vi "MU Mt Sync Calculate Position.vi"(4 "Continuous (F)":bool, 5 "Calibration Unit":u32, 6 "resolution":u64, 7 "MtTrackOffset":u8, 8 "error in (no error)":errorcluster, 9 "Samples":u64, 10 "SyncData":T1(array[cluster]), 11 "mtSyncHandle":T2) -> (0 "error out":errorcluster, 2 "MT_Position":dbl[](array[numeric]), 3 "Return Value":u64)   [LabVIEW 2017, in "MU_3SL_interface.lvlib"]
uses:
  MU_3SL_interface.lvlib
  handles/mtSyncHandle.ctl
  lib/MU_3SL_interface.dll
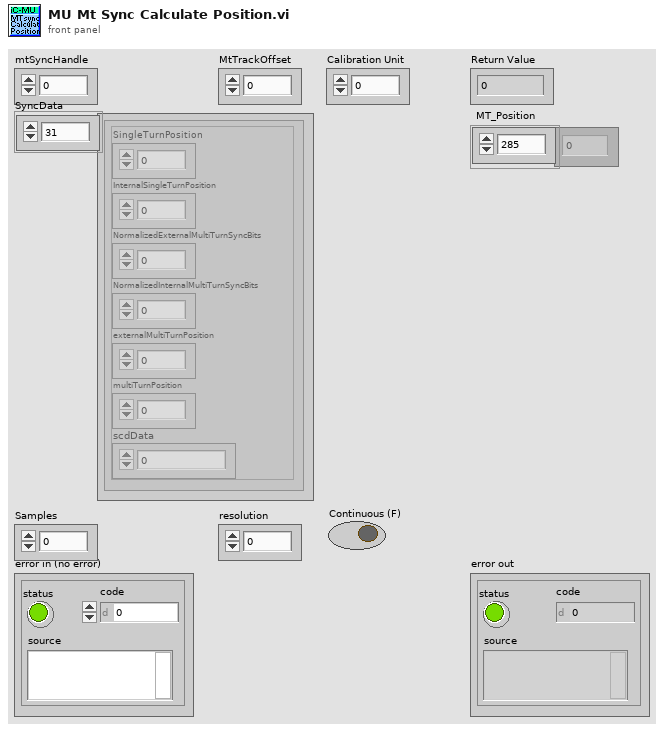
[diagram p1: front panel]
types:
  T1 = cluster{"SingleTurnPosition":u32, "InternalSingleTurnPosition":u32, "NormalizedExternalMultiTurnSyncBits":u32, "NormalizedInternalMultiTurnSyncBits":u32, "externalMultiTurnPosition":u32, "multiTurnPosition":u32, "scdData":u64}[]
  T2 = typedef "MU_3SL_interface.lvlib/mtSyncHandle.ctl" = u64
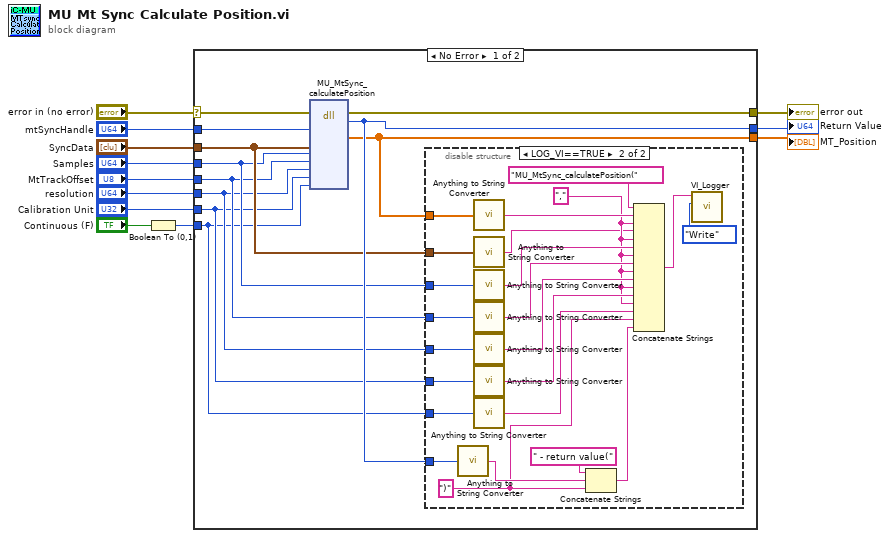
[diagram p0: block diagram]
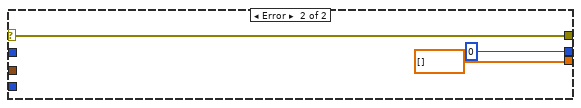
[diagram p3: hidden frame]
diagram:
  n1 = Boolean To (0,1)(Boolean="Continuous (F)") -> (0, 1=w4:i16)
  n2 = case shown="No Error" "error in (no error)" {
    selector: "error in (no error)" -> [w23 w49]
    tunnel: [w22 u64 0 ("Return Value")] -> w8
    tunnel: [w21 w49] -> w12
    tunnel: "mtSyncHandle" -> [w20 _]
    tunnel: [w19 dbl[] [] ("MT_OffsetError")] -> w9
    tunnel: "SyncData" -> [w18 _]
    tunnel: "Samples" -> [w17 _]
    tunnel: w4 -> [w13 _]
    tunnel: "resolution" -> [w15 _]
    tunnel: "MtTrackOffset" -> [w16 _]
    tunnel: "Calibration Unit" -> [w14 _]
    frame No Error {
      n3 = dll-call lib="C:/Users/bes/AppData/Roaming/work/mu_9so/icsubmodules/soft_mu_3sl_master/lv_interface/lib/MU_3SL_interface**.*" fn="MU_MtSync_calculatePosition"(error in=w23, "mtSyncHandle"=w20, "SynchronisationData"=w18, "numberOfSamples"=w17, "MtTrackOffset"=w16, "resolution"=w15, "Calibration Unit"=w14, "continuous"=w13) -> (error out=w21:errorcluster, "Return Value"=w22:u64, "MT_Position"=w19:dbl[])  [unwired: 10 in, 1 out]
      n4 = disable-structure shown="LOG_VI==TRUE" {
        disable-tunnel: w22 -> [_ w38]
        disable-tunnel: w19 -> [_ w42]
        disable-tunnel: w18 -> [_ w25]
        disable-tunnel: w17 -> [_ w40]
        disable-tunnel: w16 -> [_ w39]
        disable-tunnel: w15 -> [_ w36]
        disable-tunnel: w14 -> [_ w35]
        disable-tunnel: w13 -> [_ w34]
        frame condition #0 {
        }
        frame condition #1 (active) {
          w29 = "," ("string")
          w27 = ")" ("string")
          n5 = call "Anything to String Converter.vi"("anything"=w38) -> ("String"=w37:string)
          n6 = call "Anything to String Converter.vi"("anything"=w42) -> ("String"=w41:string)
          n7 = call "Anything to String Converter.vi"("anything"=w25) -> ("String"=w24:string)
          n8 = call "Anything to String Converter.vi"("anything"=w40) -> ("String"=w33:string)
          n9 = call "Anything to String Converter.vi"("anything"=w39) -> ("String"=w32:string)
          n10 = call "Anything to String Converter.vi"("anything"=w36) -> ("String"=w31:string)
          n11 = call "Anything to String Converter.vi"("anything"=w35) -> ("String"=w30:string)
          n12 = call "Anything to String Converter.vi"("anything"=w34) -> ("String"=w28:string)
          n13 = Concatenate Strings(" - return value(" ("string"), w37, w27) -> (w26:string)
          n14 = Concatenate Strings("MU_MtSync_calculatePosition(" ("Info in"), w41, w29, w24, w29, w33, w29, w32, w29, w31, w29, w30, w29, w28, w27, w26) -> (w44:string)
          n15 = call "VI_Logger.vi"("Action (Read)"=enum16{"Write", "Read"}."Write", "Info in"=w44) -> ()  [unwired: 8 in, 2 out]
        }
      }
    }
    frame Error {
    }
  }
  "error out" <- w12
  "MT_Position" <- w9
  "Return Value" <- w8
